vi "HelpMessage.vi"(11 "ExecuteMultipleBuildSpecs in":refnum<class "ExecuteMultipleBuildSpecs.lvclass">) -> (2 "Help":string, 3 "ExecuteMultipleBuildSpecs out":refnum<class "ExecuteMultipleBuildSpecs.lvclass">)   [LabVIEW 2014, in "ExecuteMultipleBuildSpecs.lvclass"]
doc: "The help message for this multiple build spec operation in the LabVIEWCLI."
uses:
  ExecuteMultipleBuildSpecs.lvclass
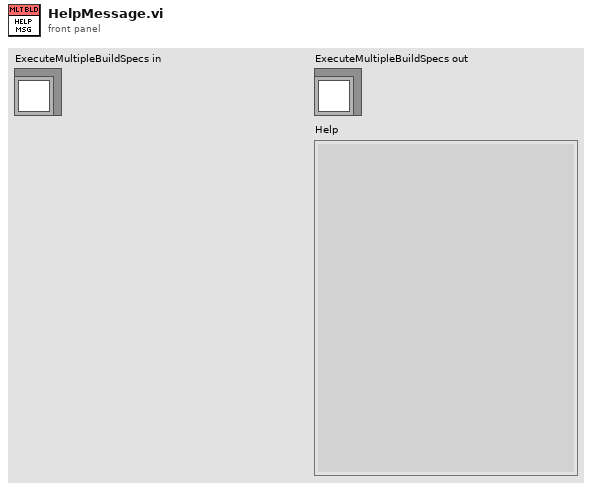
[diagram p1: front panel]
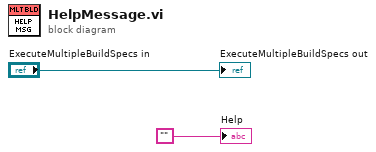
[diagram p0: block diagram]
diagram:
  "ExecuteMultipleBuildSpecs out" <- "ExecuteMultipleBuildSpecs in"
  "Help" <- ""
